vi "Camera Image Server.vi"(10 "parameters":T1(array[cluster]), 11 "connection ID":refnum<k5>) -> ()   [LabVIEW 2017, in "VisionSystem.lvlib"]
uses:
  VisionSystem.lvlib
  <vilib>/Rock Robotics/SystemInterfaces/NetworkCommunication/NetComm_UsageReport_ResourceType.ctl
  <vilib>/Rock Robotics/WPI/Camera/WPI_CameraImageSize.ctl
  <vilib>/ErrorRing/Error Ring.xnode
  <vilib>/Utility/error.llb/Error Cluster From Error Code.vi
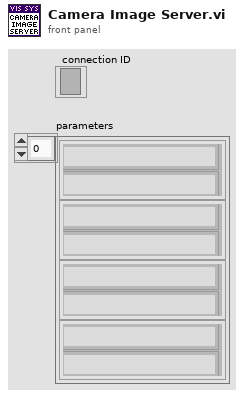
[diagram p1: front panel]
types:
  T1 = cluster{"token string":string, "token string 2":string}[]
  T2 = cluster{"White Balance":bool, "Brightness":bool, "Sharpness":bool, "Saturation":bool, "Exposure":bool}
  T3 = cluster{"White Balance":string, "Brightness":i32, "Sharpness":i32, "Saturation":i32, "Exposure":string}
  T4 = typedef "WPI_CameraImageSize.ctl" = enum16{"640x480", "320x240", "160x120", "Custom"}
  T5 = cluster{"Camera Name":string, "Size":string, "Frame Rate":i32, "Compression":i32}
  T6 = typedef "NetComm_UsageReport_ResourceType.ctl" = enum8{"Controller", "Module", "Language", "CANPlugin", "Accelerometer", "ADXL345", "AnalogChannel", "AnalogTrigger", "AnalogTriggerOutput", "CANJaguar", "Compressor", "Counter", "Dashboard", "DigitalInput", "DigitalOutput", "DriverStationCIO", "DriverStationEIO", "DriverStationLCD", "Encoder", "GearTooth", "Gyro", "I2C", "Framework", "Jaguar", "Joystick", "Kinect", "KinectStick", "PIDController", "Preferences", "PWM", "Relay", "RobotDrive", "SerialPort", "Servo", "Solenoid", "SPI", "Task", "Ultrasonic", "Victor", "Button", "Command", "AxisCamera", "PCVideoServer", "SmartDashboard", "Talon", "HiTechnicColorSensor", "HiTechnicAccel", "HiTechnicCompass", "SRF08", "AnalogOutput", "Victor SP", "Talon SRX", "CAN Talon SRX", "ADXL362 Accel", "ADXRS450 Gyro", "Rev SPARK", "Mindsensors SD540", "Digital Filter", "ADIS16448", "PDP", "PCM", "PigeonIMU", "Nidec Brushless", "CTRE CANifier", "CTRE Future 0", "CTRE Future 1", "CTRE Future 2", "CTRE Future 3", "CTRE Future 4", "CTRE Future 5", "CTRE Future 6"}
  T7 = typedef "WPI_CameraDevRef.ctl" = cluster{"Camera Address":string, "CameraStatus":errorcluster}
  T8 = typedef "WPI_CameraWhite Balance Values.ctl" = enum16{"Auto", "Fixed indoor", "Fixed outdoor 1", "Fixed outdoor 2", "Fixed fluorescent 1", "Fixed fluorescent 2", "Hold current", "Custom"}
  T9 = typedef "WPI_CameraExposure Values.ctl" = enum16{"Auto", "Flicker-free 50 Hz", "Flicker-free 60 Hz", "Hold current", "Custom"}
  T10 = enum16{"Update Mode", "Get Image", "Get Image Data"}
  T11 = typedef "Image Type" = u32
  T12 = typedef "IMAQ Image.ctl" = refnum<image>
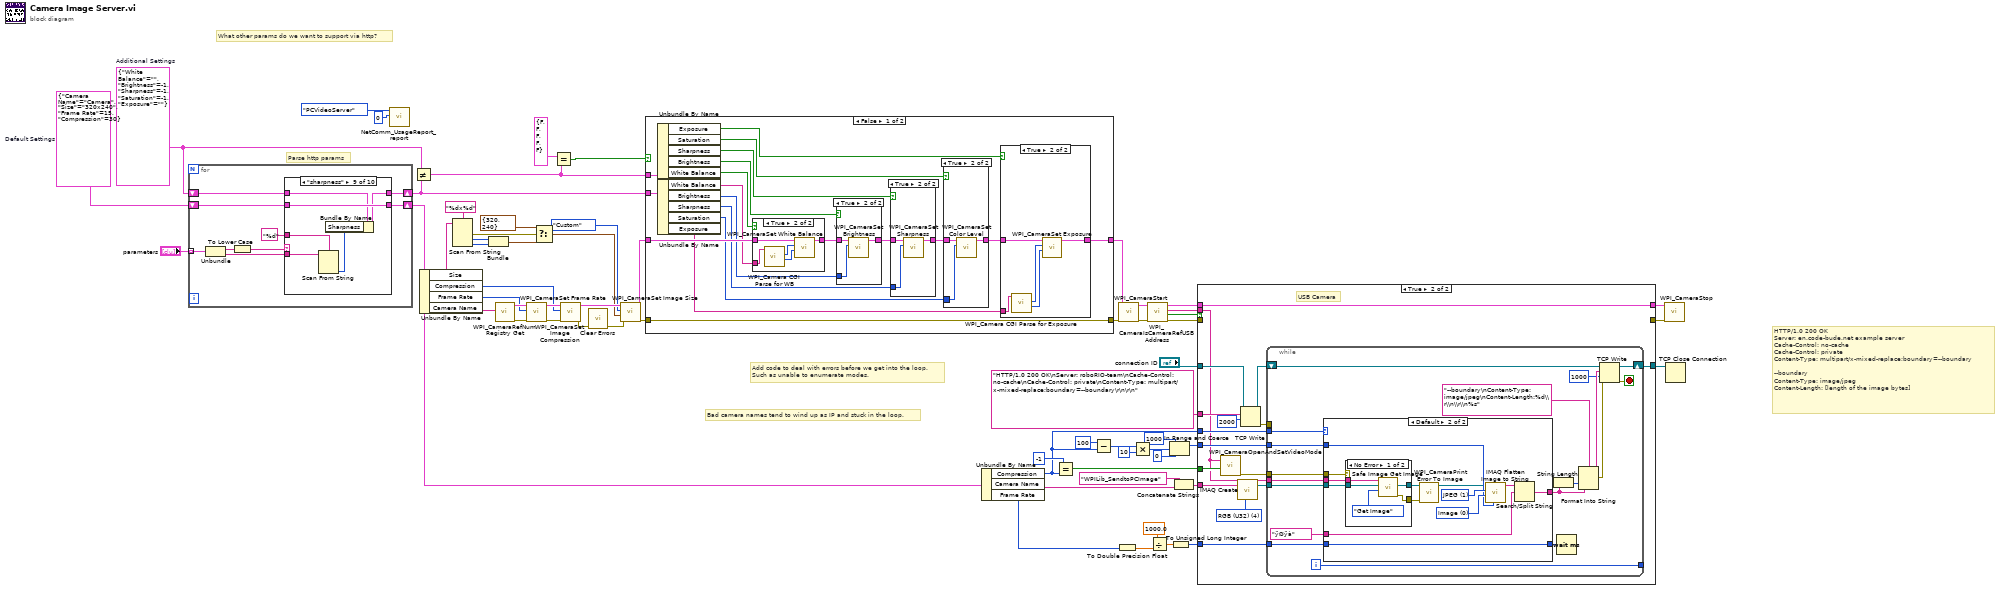
[diagram p0: block diagram]
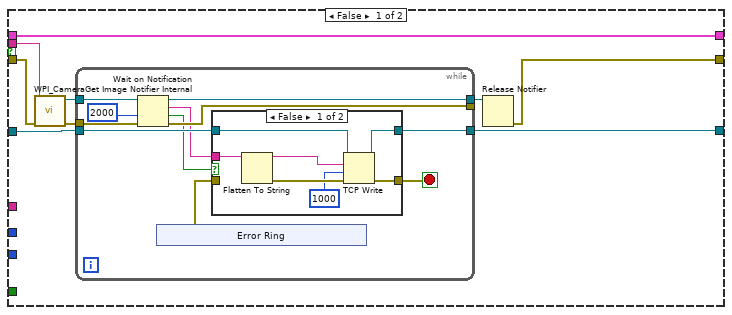
[diagram p8: hidden frame]
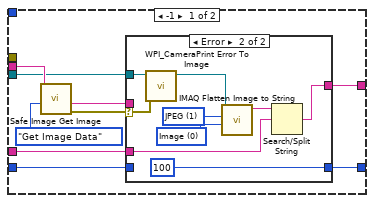
[diagram p10: hidden frame]
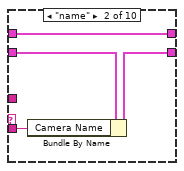
[diagram p14: hidden frame]
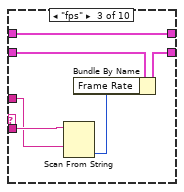
[diagram p15: hidden frame]
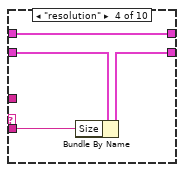
[diagram p16: hidden frame]
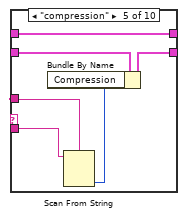
[diagram p17: hidden frame]
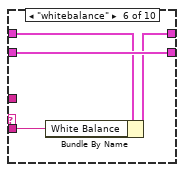
[diagram p18: hidden frame]
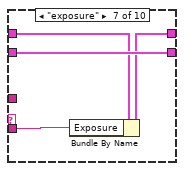
[diagram p19: hidden frame]
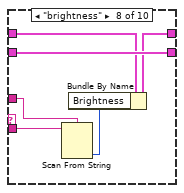
[diagram p20: hidden frame]
diagram:
  w18 = T3 {"White Balance"="", "Brightness"=-1, "Sharpness"=-1, "Saturation"=-1, "Exposure"=""}  # Additional Settings
  w59 = T5 {"Camera Name"="Camera", "Size"="320x240", "Frame Rate"=15, "Compression"=30}  # Default Settings
  # "Add code to deal with errors before we get into the loop.\nSuch as unable to enumerate modes."
  # "Parse http params"
  # "Bad camera names tend to wind up as IP and stuck in the loop."
  # "What other params do we want to support via http?"
  # "HTTP/1.0 200 OK\nServer: en.code-bude.net example server\nCache-Control: no-cache\nCache-Control: private\nContent-Type: multipart/x-mixed-replace;boundary=--boundary\n \n--boundary\nContent-Type: image/jpeg\nContent-Length: [length of the image bytes]"
  n1 = for {
    tunnel: "parameters" -> [w71] mode=indexing
    shift-right: [w66] -> w7
    shift-left: w59 -> [w68]
    shift-right: [w63] -> w12
    shift-left: w18 -> [w64]
    n2 = Unbundle(w71) -> ("token string"=w70:string, "token string 2"=w67:string)
    n3 = To Lower Case(string=w70) -> (all lower case string=w69:string)
    n4 = case shown="\"sharpness\"" w69 {
      tunnel: w68 -> [w73 w77 w83 w87 w93 w97 w101 w107 w113 w119]
      tunnel: w67 -> [_ w76 w81 w85 w91 w95 w98 w103 w109 w115]
      tunnel: [w73 w75 w82 w86 w92 w97 w101 w107 w113 w119] -> w66
      tunnel: "%d" -> [_ _ w80 _ w89 _ _ w104 w110 w116]
      tunnel: w64 -> [w72 w74 w78 w84 w88 w96 w100 w106 w112 w118]
      tunnel: [w72 w74 w78 w84 w88 w94 w99 w105 w111 w117] -> w63
      frame Default {
      }
      frame "name" {
        n5 = Bundle By Name(cluster=w77, "Camera Name"=w76) -> (w75:T5)
      }
      frame "fps" {
        n6 = Scan From String(format string=w80, input string=w81) -> (output 1=w79:i32)  [unwired: 3 in, 3 out]
        n7 = Bundle By Name(cluster=w83, "Frame Rate"=w79) -> (w82:T5)
      }
      frame "resolution" {
        n8 = Bundle By Name(cluster=w87, "Size"=w85) -> (w86:T5)
      }
      frame "compression" {
        n9 = Scan From String(format string=w89, input string=w91) -> (output 1=w90:i32)  [unwired: 3 in, 3 out]
        n10 = Bundle By Name(cluster=w93, "Compression"=w90) -> (w92:T5)
      }
      frame "whitebalance" {
        n11 = Bundle By Name(cluster=w96, "White Balance"=w95) -> (w94:T3)
      }
      frame "exposure" {
        n12 = Bundle By Name(cluster=w100, "Exposure"=w98) -> (w99:T3)
      }
      frame "brightness" {
        n13 = Scan From String(format string=w104, input string=w103) -> (output 1=w102:i32)  [unwired: 3 in, 3 out]
        n14 = Bundle By Name(cluster=w106, "Brightness"=w102) -> (w105:T3)
      }
      frame "sharpness" {
        n15 = Scan From String(format string=w110, input string=w109) -> (output 1=w108:i32)  [unwired: 3 in, 3 out]
        n16 = Bundle By Name(cluster=w112, "Sharpness"=w108) -> (w111:T3)
      }
      frame "colorlevel" {
        n17 = Scan From String(format string=w116, input string=w115) -> (output 1=w114:i32)  [unwired: 3 in, 3 out]
        n18 = Bundle By Name(cluster=w118, "Saturation"=w114) -> (w117:T3)
      }
    }
  }
  n19 = call <vilib>:"NetComm_UsageReport_report.vi"("Instance Number"=u8 0, "Resource Type"=NetComm_UsageReport_ResourceType."PCVideoServer") -> ()  [unwired: 10 in]
  n20 = Not Equal?(x=w18, y=w12) -> (x != y?=w15:T2)
  n21 = Unbundle By Name(w7) -> ("Size"=w31:string, "Compression"=w6:i32, "Frame Rate"=w2:i32, "Camera Name"=w4:string)
  n22 = Scan From String(format string="%dx%d", input string=w31) -> (error out=w26:errorcluster, output 1=w29:i32, output 2=w28:i32)  [unwired: 4 in, 2 out]
  n23 = Bundle(w29, w28) -> (w25:cluster{i32, i32})  [unwired: 1 in]
  n24 = call <vilib>:"WPI_CameraRefNum Registry Get.vi"("refnum name"=w4) -> ("error out"=w32:errorcluster, "CameraDevRef"=w33:T7)  [unwired: 9 in]
  n25 = call <vilib>:"WPI_CameraSet Frame Rate.vi"("error in (no error)"=w32, "Frame Rate (fps)"=w2, "CameraDevRef"=w33) -> ("error out"=w47:errorcluster, "CameraDevRef Out"=w49:T7)  [unwired: 7 in]
  n26 = Select(t=cluster{i32, i32} {320, 240} ("s? t:f"), s=w26, f=w25) -> (s? t:f=w24:cluster{i32, i32})
  n27 = Equal?(x=T2 {"White Balance"=FALSE, "Brightness"=FALSE, "Sharpness"=FALSE, "Saturation"=FALSE, "Exposure"=FALSE} ("x != y?"), y=w15) -> (x = y?=w16:bool)
  n28 = call <vilib>:"WPI_CameraSet Image Compression.vi"("error in (no error)"=w47, "Compression"=w6, "CameraDevRef"=w49) -> ("error out"=w35:errorcluster, "CameraDevRef Out"=w48:T7)  [unwired: 7 in]
  n29 = call <vilib>:"Clear Errors.vi"("error in (no error)"=w35) -> ("error out"=w34:errorcluster)  [unwired: 5 in, 1 out]
  n30 = call <vilib>:"WPI_CameraSet Image Size.vi"("error in (no error)"=w34, "Size W,H (pix)"=w24, "Image Size"=WPI_CameraImageSize."Custom", "CameraDevRef"=w48) -> ("error out"=w10:errorcluster, "CameraDevRef Out"=w14:T7)  [unwired: 6 in]
  n31 = case shown="False" w16 {
    tunnel: w15 -> [w138 _]
    tunnel: w14 -> [w136 w164]
    tunnel: [w131 w164] -> w13
    tunnel: w12 -> [w130 _]
    tunnel: w10 -> [w124 w163]
    tunnel: [w124 w163] -> w9
    frame False {
      n32 = Unbundle By Name(w138) -> ("Exposure"=w120:bool, "Saturation"=w137:bool, "Sharpness"=w121:bool, "Brightness"=w122:bool, "White Balance"=w123:bool)
      n33 = Unbundle By Name(w130) -> ("White Balance"=w129:string, "Brightness"=w128:i32, "Sharpness"=w127:i32, "Saturation"=w126:i32, "Exposure"=w125:string)
      n34 = case shown="True" w123 {
        tunnel: w136 -> [w157 w162]
        tunnel: [w157 w161] -> w135
        tunnel: w129 -> [_ w158]
        frame False {
        }
        frame True {
          n35 = call <vilib>:"WPI_Camera CGI Parse for WB.vi"("String"=w158) -> ("Numeric"=w159:i32, "enum"=w160:T8)  [unwired: 9 in]
          n36 = call <vilib>:"WPI_CameraSet White Balance.vi"("Color Temp (K)"=w159, "White Balance"=w160, "CameraDevRef"=w162) -> ("CameraDevRef Out"=w161:T7)  [unwired: 7 in, 1 out]
        }
      }
      n37 = case shown="True" w122 {
        tunnel: w135 -> [w153 w156]
        tunnel: [w153 w155] -> w134
        tunnel: w128 -> [_ w154]
        frame False {
        }
        frame True {
          n38 = call <vilib>:"WPI_CameraSet Brightness.vi"("Brightness"=w154, "CameraDevRef"=w156) -> ("CameraDevRef Out"=w155:T7)  [unwired: 8 in, 1 out]
        }
      }
      n39 = case shown="True" w121 {
        tunnel: w134 -> [w149 w152]
        tunnel: [w149 w151] -> w133
        tunnel: w127 -> [_ w150]
        frame False {
        }
        frame True {
          n40 = call <vilib>:"WPI_CameraSet Sharpness.vi"("Sharpness"=w150, "CameraDevRef"=w152) -> ("CameraDevRef Out"=w151:T7)  [unwired: 8 in, 1 out]
        }
      }
      n41 = case shown="True" w137 {
        tunnel: w133 -> [w145 w148]
        tunnel: [w145 w147] -> w132
        tunnel: w126 -> [_ w146]
        frame False {
        }
        frame True {
          n42 = call <vilib>:"WPI_CameraSet Color Level.vi"("Color Level"=w146, "CameraDevRef"=w148) -> ("CameraDevRef Out"=w147:T7)  [unwired: 8 in, 1 out]
        }
      }
      n43 = case shown="True" w120 {
        tunnel: w132 -> [w139 w144]
        tunnel: [w139 w143] -> w131
        tunnel: w125 -> [_ w142]
        frame False {
        }
        frame True {
          n44 = call <vilib>:"WPI_Camera CGI Parse for Exposure.vi"("String"=w142) -> ("Numeric"=w141:i32, "enum"=w140:T9)  [unwired: 9 in]
          n45 = call <vilib>:"WPI_CameraSet Exposure.vi"("Exposure (%)"=w141, "Exposure"=w140, "CameraDevRef"=w144) -> ("CameraDevRef Out"=w143:T7)  [unwired: 7 in, 1 out]
        }
      }
    }
    frame True {
      # "Unchanged, none to set"
    }
  }
  n46 = Unbundle By Name(w7) -> ("Compression"=w5:i32, "Camera Name"=w3:string, "Frame Rate"=w1:i32)
  n47 = Equal?(x=-1, y=w5) -> (x = y?=w36:bool)
  n48 = Subtract(x=100, y=w5) -> (x-y=w40:i32)
  n49 = To Double Precision Float(number=w1) -> (double precision float=w11:dbl)
  n50 = call <vilib>:"WPI_CameraStart.vi"("error in (no error)"=w9, "CameraDevRef"=w13) -> ("error out"=w52:errorcluster, "CameraDevRef"=w51:T7)  [unwired: 8 out]
  n51 = Multiply(x=w40, y=10) -> (x*y=w42:i32)
  n52 = call <vilib>:"WPI_CameraIsCameraRefUSBAddress.vi"("error in (no error)"=w52, "CameraDevRef"=w51) -> ("error out"=w22:errorcluster, "USB?"=w53:bool, "Camera Address Out"=w54:string, "CameraDevRef out"=w50:T7)  [unwired: 6 in]
  n53 = Divide(x=1000.0 ("port"), y=w11) -> (x/y=w45:dbl)
  n54 = In Range and Coerce(upper limit=1000, x=w42, lower limit=0) -> (coerced(x)=w38:i32)  [unwired: 1 out]
  n55 = To Unsigned Long Integer(number=w45) -> (unsigned 32bit integer=w8:u32)
  n56 = Concatenate Strings("WPILib_SendtoPCImage", w3) -> (w19:string)
  n57 = case shown="True" w53 {
    tunnel: "connection ID" -> [w173 w206]
    tunnel: [w172 w213] -> w62
    tunnel: w22 -> [w171 _]
    tunnel: w54 -> [w169 w199]
    tunnel: [w165 w198] -> w56
    tunnel: w50 -> [w165 w198]
    tunnel: [w167 _] -> w55
    tunnel: w19 -> [_ w211]
    tunnel: w38 -> [_ w207]
    tunnel: w8 -> [_ w210]
    tunnel: w5 -> [_ w209]
    tunnel: w36 -> [_ w208]
    tunnel: "HTTP/1.0 200 OK\nServer: roboRIO-team\nCache-Control: no-cache\nCache-Control: private\nContent-Type: multipart/x-mixed-replace;boundary=--boundary\r\n\r\n" ("regular expression") -> [_ w203]
    frame False {
      n58 = call <vilib>:"WPI_CameraGet Image Notifier Internal.vi"("error in (no error)"=w171, "Camera Address"=w169) -> ("error out"=w170:errorcluster, "Image Notifier"=w168:refnum<notifier>)  [unwired: 8 out]
      n59 = while {
        tunnel: w170 -> [w184]
        tunnel: w173 -> [w180]
        tunnel: [w182] -> _
        tunnel: [w179] -> w172
        tunnel: w168 -> [w183]
        tunnel: [w181] -> w166
        stop <- w176 stop-if-true
        n60 = Wait on Notification(notifier=w183, timeout in ms (-1)=2000 ("Timeout in ms (-1)"), error in (no error)=w184) -> (notifier out=w181:refnum<notifier>, notification=w178:string, timed out?=w177:bool, error out=w182:errorcluster)  [unwired: 1 out]
        n61 = xnode "Error Ring"() -> ("error out"=w175:errorcluster)
        n62 = case shown="False" w177 {
          tunnel: [w189 w192] -> w176
          tunnel: w180 -> [w188 w193]
          tunnel: [w186 w193] -> w179
          tunnel: w178 -> [w187 _]
          tunnel: w175 -> [_ w192]
          frame False {
            n63 = Flatten To String(anything=w187) -> (data string=w191:string, error out=w190:errorcluster)  [unwired: 1 in, 3 out]
            n64 = TCP Write(connection ID=w188, data in=w191, error in (no error)=w190, 9:1000 ("timeout ms (25000)")) -> (connection ID out=w186:refnum<k5>, error out=w189:errorcluster)  [unwired: 1 out]
          }
          frame True {
          }
        }
      }
      n65 = Release Notifier(notifier=w166) -> (error out=w167:errorcluster)  [unwired: 1 in, 3 out]
    }
    frame True {
      w200 = T11 4 items=["Grayscale (U8)", "Grayscale (I16)", "Grayscale (SGL)", "Complex (CSG)", "RGB (U32)", "HSL (U32)", "RGB (U64)", "Grayscale (U16)"] ("Image Type")
      # "USB Camera"
      n66 = call <vilib>:"WPI_CameraOpenAndSetVideoMode.vi"("USB JPEG"=w208, "Camera Address"=w199) -> ("error out"=w201:errorcluster)  [unwired: 9 in]
      n67 = call "IMAQ Create"("Image Name"=w211, "Image Type"=w200) -> ("New Image"=w212:T12)  [unwired: 3 in, 1 out]
      n68 = TCP Write(connection ID=w206, data in=w203, 9:2000) -> (connection ID out=w205:refnum<k5>, error out=w204:errorcluster)  [unwired: 1 in, 1 out]
      n69 = while {
        tunnel: w199 -> [w231]
        shift-right: [w219] -> w213
        shift-left: w205 -> [w215]
        tunnel: w212 -> [w230]
        tunnel: w210 -> [w217]
        tunnel: w209 -> [w229]
        tunnel: w204 -> [_]
        tunnel: w207 -> [w228]
        tunnel: [w221] -> _
        tunnel: w201 -> [w218]
        i -> [w221]
        stop <- w220 stop-if-true
        n70 = case shown="Default" w229 {
          tunnel: [w237 w258] -> w225
          tunnel: w231 -> [w240 w261]
          tunnel: w230 -> [w236 w260]
          tunnel: w228 -> [_ w262]
          tunnel: "ÿØÿà" ("format string") -> [w235 w259]
          tunnel: w218 -> [_ w255]
          tunnel: w217 -> [w234 w252]
          tunnel: [w233 w252] -> w216
          frame -1 {
            n71 = call <vilib>:"Safe Image Get Image.vi"("Operation"=T10."Get Image Data", "Session In"=w240) -> ("error out"=w239:errorcluster, "Image Data String"=w238:string)  [unwired: 6 in, 2 out]
            n72 = case shown="Error" w239 {
              selector: w239 -> [_ w251]
              tunnel: [w242 w244] -> w237
              tunnel: w238 -> [w242 _]
              tunnel: w236 -> [_ w248]
              tunnel: w235 -> [_ w246]
              tunnel: w234 -> [w241 _]
              tunnel: [w241 u32 100 ("port")] -> w233
              frame No Error {
              }
              frame Error {
                w249 = 0 items=["Image", "Image and Vision Info", "Reference to Image"] ("Type of Flatten (Image and Vision Info)")
                w250 = 1 items=["None", "JPEG", "PACKED BINARY"] ("Compression (None)")
                n73 = call <vilib>:"WPI_CameraPrint Error To Image.vi"("error in (no error)"=w251, "Image"=w248) -> ("Image out"=w247:T12)  [unwired: 8 in, 1 out]
                n74 = call "IMAQ Flatten Image to String"("Type of Flatten (Image and Vision Info)"=w249, "Compression (None)"=w250, "Image"=w247) -> ("Data String"=w245:string)  [unwired: 7 in, 1 out]
                n75 = Search/Split String(string=w245, search string/char (-)=w246) -> (match + rest of string=w244:string)  [unwired: 1 in, 2 out]
              }
            }
          }
          frame Default {
            w263 = 0 items=["Image", "Image and Vision Info", "Reference to Image"] ("Type of Flatten (Image and Vision Info)")
            w264 = 1 items=["None", "JPEG", "PACKED BINARY"] ("Compression (None)")
            n76 = case shown="No Error" w255 {
              selector: w255 -> [_ w270]
              tunnel: w261 -> [w269 _]
              tunnel: w260 -> [w268 w271]
              tunnel: [w267 w270] -> w257
              tunnel: [w266 w271] -> w256
              frame No Error {
                n77 = call <vilib>:"Safe Image Get Image.vi"("Operation"=T10."Get Image", "Image In"=w268, "Session In"=w269) -> ("error out"=w267:errorcluster, "Image Out"=w266:T12)  [unwired: 5 in, 2 out]
              }
              frame Error {
              }
            }
            n78 = call <vilib>:"WPI_CameraPrint Error To Image.vi"("error in (no error)"=w257, "Image"=w256) -> ("Image out"=w253:T12)  [unwired: 8 in, 1 out]
            n79 = call "IMAQ Flatten Image to String"("Quality (750)"=w262, "Type of Flatten (Image and Vision Info)"=w263, "Compression (None)"=w264, "Image"=w253) -> ("Data String"=w254:string)  [unwired: 6 in, 1 out]
            n80 = Search/Split String(string=w254, search string/char (-)=w259) -> (match + rest of string=w258:string)  [unwired: 1 in, 2 out]
          }
        }
        n81 = String Length(string=w225) -> (length=w226:i32)
        n82 = Wait (ms)(milliseconds to wait=w216) -> ()  [unwired: 1 out]
        n83 = Format Into String(format string="--boundary\nContent-Type: image/jpeg\nContent-Length:%d\\r\\n\\r\\n%s" ("regular expression"), w226, w225) -> (resulting string=w223:string, error out=w224:errorcluster)  [unwired: 2 in]
        n84 = TCP Write(connection ID=w215, data in=w223, error in (no error)=w224, 9:1000 ("timeout ms (25000)")) -> (connection ID out=w219:refnum<k5>, error out=w220:errorcluster)  [unwired: 1 out]
      }
    }
  }
  n85 = call <vilib>:"WPI_CameraStop.vi"("error in (no error)"=w55, "CameraDevRef"=w56) -> ()  [unwired: 10 out]
  n86 = TCP Close Connection(connection ID=w62) -> ()  [unwired: 1 in, 3 out]
